vi "Pre Launch Init.vi"(11 "DAQ Actor in":refnum<class "DAQ Actor.lvclass">) -> (0 "error out":errorcluster, 3 "DAQ Actor out":refnum<class "DAQ Actor.lvclass">)   [LabVIEW 2017, in "DAQ Actor.lvlib" / "DAQ Actor.lvclass"]
doc: "(<B>Filename</B>: Actor Framework.lvlib:Actor.lvclass:Pre Launch Init.vi)\n\nDefines behavior that occurs after the Launch Nested Actor method is invoked but before the actor's Actor Core method begins running.\n\nBy default, this method does nothing. A descendant class may override it to define behavior."
uses:
  DAQ Actor.lvclass
  DAQ Actor.lvclass/DAQ Actor.ctl
  <vilib>/DAQmx/create/channels.llb/DAQmx Create Channel (AI-Voltage-Basic).vi
  <vilib>/ActorFramework/Actor/Actor.lvclass
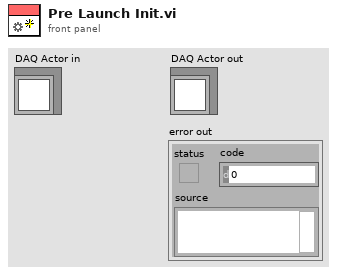
[diagram p1: front panel]
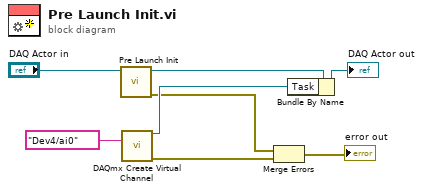
[diagram p0: block diagram]
diagram:
  n1 = call-parent "Pre Launch Init.vi"("Actor in"="DAQ Actor in") -> ("error out"=w3:errorcluster, "Actor out"=w8:refnum<class "DAQ Actor.lvclass">)  [unwired: 9 in]
  n2 = call-poly <vilib>:"DAQmx Create Virtual Channel.vi"("physical channels"=tag "Dev4/ai0") -> ("task out"=w5:refnum<k21>, "error out"=w2:errorcluster)  [unwired: 13 in]
  n3 = Merge Errors(w3, w2) -> (→"error out":errorcluster)
  n4 = Bundle By Name(cluster=w8, "Task"=w5) -> (→"DAQ Actor out":refnum<class "DAQ Actor.lvclass">)
